vi "自动测试结果.vi"() -> ()   [LabVIEW 2010]
panel:
  out "Auto_LAN_R":bool
  in  "Auto_RS485_R":bool[](array[boolean])
  in  "Auto_RS232_R":bool[](array[boolean])
  in  "Auto_CAN_R":bool[](array[boolean])
  out "自测总概述":string
  out "串口RS485测试概述":string
  out "模拟量DSP概述":string
  in  "Auto_AD_max_WC":dbl[](array[numeric]) format="%#.4f"
  in  "Auto_DSP_max_WC":dbl[](array[numeric]) format="%#.4f"
  in  "总线通信自测结果":string[][](array[string])
  in  "AI自动测试结果":string[][](array[string])
  in  "DO自动测试结果":string[][](array[string])
  in  "Auto_AD_R":bool[](array[boolean])
  in  "Auto_DSP_R":bool[](array[boolean])
  in  "Auto_DO_R":bool[][](array[boolean])
  in  "Auto_DI_R":bool[][](array[boolean])
  in  "DI自动测试结果":string[][](array[string])
  out "以太网测试概述":string
  out "串口RS232测试概述":string
  out "CAN测试概述":string
  out "模拟量AD概述结果":string
  out "数字量输出概述":string
  out "数字量输入概述":string
  in  "Auto_COM_Reault":string[](array[string])
  in  "Auto_COM_Back":string[](array[string])
  in  "Auto_COM_In":string[](array[string])
  in  "Auto_DO_Table":string[][](array[string])
  in  "Auto_DI_Table":string[][](array[string])
  in  "Auto_AI_AD_WC":string[][](array[string])
  in  "Auto_AI_AD_Back":string[][](array[string])
  in  "Auto_AI_AD_IN":string[][](array[string])
  in  "Auto_AI_PWM_WC":string[][](array[string])
  in  "Auto_AI_PWM_Back":string[][](array[string])
  in  "Auto_AI_PWM_IN":string[][](array[string])
  in  "Auto_DO_Back":string[][][](array[string])
  in  "Auto_DI_Result":string[][][](array[string])
  in  "Auto_DO_Result":string[][][](array[string])
  in  "Auto_DI_Back":string[][][](array[string])
  # "2X5X16"
  # "80X7"
  # "2X5X16"
  # "2X5X16"
  # "2X5X16"
  # "80X7"
  # "16X5"
  # "16X5"
  # "16X5"
  # "16X5"
  # "16X5"
  # "16X5"
  # "1X3"
  # "1X3"
  # "1X3"
  # "自动测试"
  # "共测多类项"
  # "nx3"
  # "nx3"
  # "nx4"
  # "nx3"
  # "5X16"
  # "自动测试数字量输入最终结论 0和1综合后结论"
  # "5X16"
  # "自动测试数字量输出最终结论 0和1综合后结论"
  # "自动测试模拟量DSP输入最终结论 5组综合后结论"
  # "1X16"
  # "1X16"
  # "自动测试模拟量AD输入最终结论 5组综合后结论"
  # "1X16"
  # "自动测试模拟量DSP最大误差"
  # "1X16"
  # "自动测试模拟量AD最大误差"
  # "1X4"
  # "1X2"
  # "1X1"
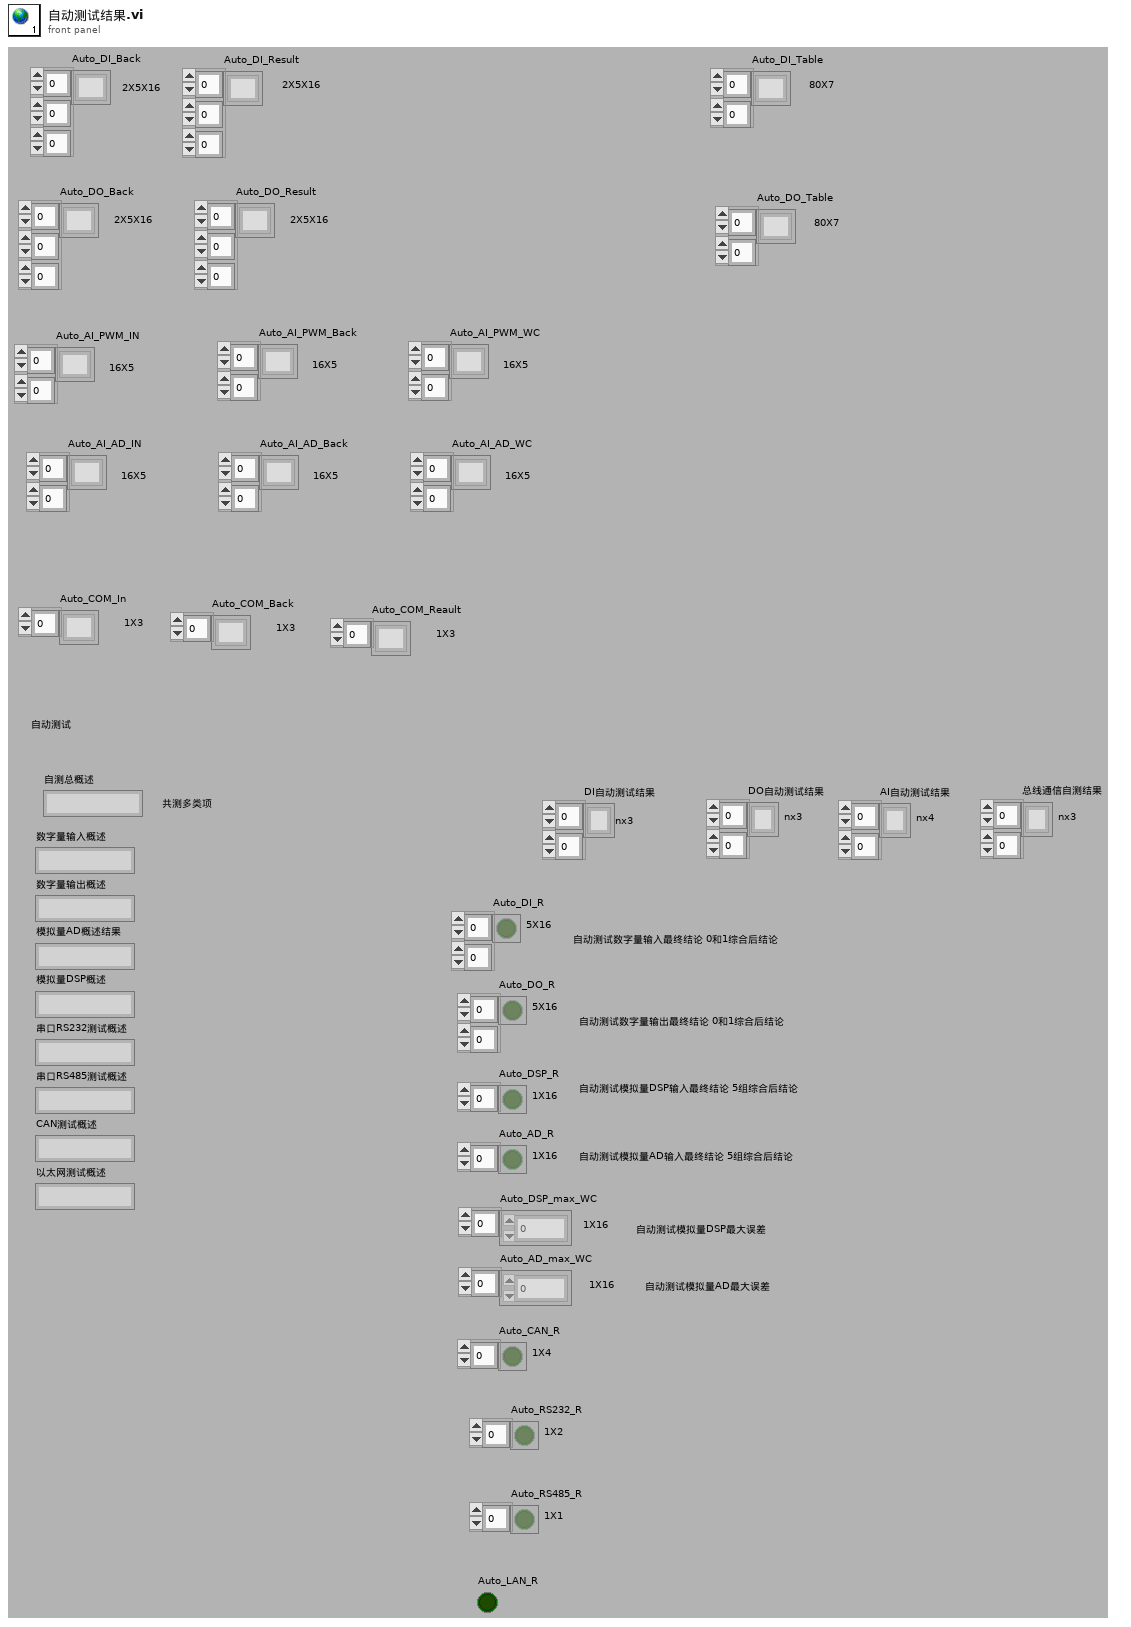
[diagram p1: front panel]
diagram:
